vi "get FPGA CD resources.vi"(8 "error in (no error)":errorcluster, 9 "get unmapped?":bool, 10 "get mapped?":bool, 11 "Item Ref in":T2 format="%.0x") -> (0 "error out":errorcluster, 3 "FPGA CD resources":T1[](array[typedef]) {"FPGA CD Ref" format="%.0x"; "reserver" format="%.0x"})   [LabVIEW 2016, in "FPGA Resource Manager System Defintion.lvlib"]
uses:
  FPGA Resource Manager System Defintion.lvlib
  <vilib>/NI Veristand/Custom Device API/Custom Device Item Ref.ctl
  resource info.ctl
  FPGA-Addon/Source/Shared/FG Action.ctl
  global constants.vi
  <vilib>/NI Veristand/Custom Device API/NI VeriStand - Get Item Property.vi
  <vilib>/NI Veristand/Custom Device API/Get Item Property (Variant).vi
  <vilib>/NI Veristand/Custom Device API/NI VeriStand - Set Item Property.vi
  <vilib>/NI Veristand/Custom Device API/Set Item Property (Variant).vi
  <vilib>/NI Veristand/Custom Device API/Custom Device API.lvlib
  FPGA Resource Manager Shared.lvlib
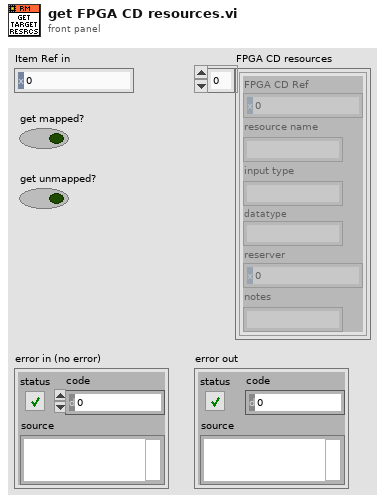
[diagram p1: front panel]
types:
  T1 = typedef "FPGA Resource Manager System Defintion.lvlib/resource info.ctl" = cluster{"FPGA CD Ref":T2, "resource name":string, "input type":string, "datatype":string, "reserver":T2, "notes":string}
  T2 = typedef "Custom Device API.lvlib/Custom Device Item Ref.ctl" = u64
  T3 = typedef "FPGA Resource Manager Shared.lvlib/FG Action.ctl" = enum8{"GET", "SET"}
  T4 = typedef "Custom Device API.lvlib/Custom Device Item Info.ctl" = cluster{"Name":string, "Is Channel":bool, "GUID":string, "Is Waveform":bool}
  T5 = typedef "FPGA Addon Shared.lvlib/Register Information.ctl" = cluster{"Name":string, "Data Type":T6, "Default Value":variant}
  T6 = typedef "FPGA Addon Shared.lvlib/Data Type.ctl" = enum8{"<Null>", "I8", "I16", "I32", "I64", "U8", "U16", "U32", "U64", "SGL", "Boolean", "Analog PWM In Settings", "Analog PWM In", "Digital PWM In Settings", "Digital PWM In", "Digital PWM Out", "Sine Out", "FXP+/-24.5", "FXP+/-16.5", "FXP+/-32.8", "FXP+/-64.32", "FXP+/-16.7", "FXP+/-20.5"}
  T7 = typedef "Fifo_DMA_Config.ctl" = cluster{"Name":string, "Depth":u32, "Write? (Deprecated:Use Implementation)":bool, "Physical Channel":u32, "Base Address":u32, "Data Width":u32, "Data Type":T8, "FXP Properties":variant, "Write Window Address":u32, "Implementation":T9, "Control Set":u32}
  T8 = typedef "niFpgaDataTypeControl.ctl" = enum32{"Boolean", "I8", "I16", "I32", "I64", "U8", "U16", "U32", "U64", "FXP", "CustomControl", "SGL"}
  T9 = typedef "niFpgaDmaChannelImplementation.ctl" = enum16{"niFpgaTargetToHost", "niFpgaHostToTarget", "niFpgaPeerToPeerWriter", "niFpgaPeerToPeerReader", "niCoreTargetToHost", "niCoreHostToTarget"}
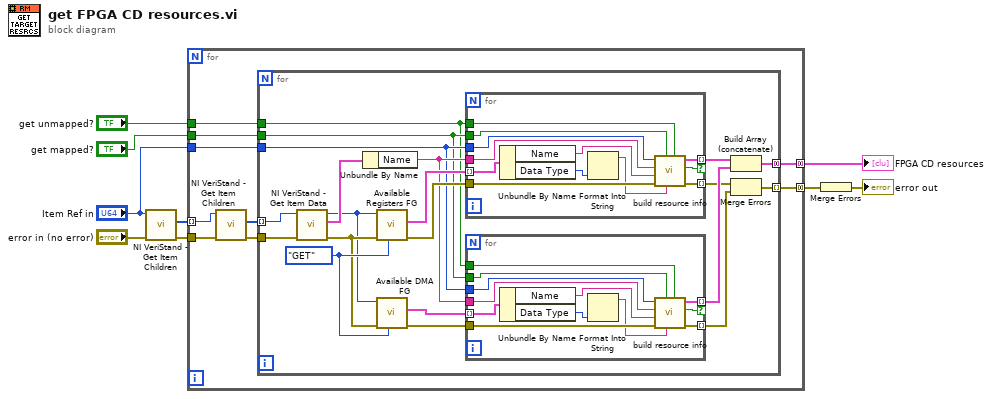
[diagram p0: block diagram]
diagram:
  n1 = call <vilib>:"NI VeriStand - Get Item Children.vi"("error in (no error)"="error in (no error)", "Item Ref in"="Item Ref in") -> ("error out"=w5:errorcluster, "Child Refs"=w6:T2[])  [unwired: 6 in, 2 out]
  n2 = for {
    tunnel: w5 -> [w17]
    tunnel: w6 -> [w15] mode=indexing
    tunnel: "Item Ref in" -> [w14]
    tunnel: [w13] -> w7 mode=concatenating
    tunnel: [w12] -> w2 mode=concatenating
    tunnel: "get mapped?" -> [w11]
    tunnel: "get unmapped?" -> [w10]
    n3 = call <vilib>:"NI VeriStand - Get Item Children.vi"("error in (no error)"=w17, "Item Ref in"=w15) -> ("error out"=w16:errorcluster, "Child Refs"=w18:T2[])  [unwired: 6 in, 2 out]
    n4 = for {
      tunnel: w16 -> [w29]
      tunnel: w18 -> [w32] mode=indexing
      tunnel: w14 -> [w23]
      tunnel: [w36] -> w13 mode=indexing
      tunnel: [w34] -> w12 mode=concatenating
      tunnel: w11 -> [w22]
      tunnel: w10 -> [w21]
      w33 = FG_Action."GET" ("Action")
      n5 = call <vilib>:"NI VeriStand - Get Item Data.vi"("error in (no error)"=w29, "Item Ref in"=w32) -> ("error out"=w28:errorcluster, "Item Info"=w31:T4, "Item Ref out"=w27:T2)  [unwired: 6 in, 1 out]
      n6 = Unbundle By Name(w31) -> ("Name"=w24:string)
      n7 = call "Available Registers FG.vi"("Action"=w33, "error in (no error)"=w28, "Item Ref"=w27) -> ("error out"=w25:errorcluster, "Available Registers"=w26:T5[])  [unwired: 6 in, 1 out]
      n8 = call "Available DMA FG.vi"("Action"=w33, "error in (no error)"=w28, "Item Ref"=w27) -> ("error out"=w30:errorcluster, "Available DMA"=w38:T7[])  [unwired: 6 in, 1 out]
      n9 = for {
        tunnel: w26 -> [w50] mode=indexing
        tunnel: w25 -> [w48]
        tunnel: [w47] -> w19 mode=indexing
        tunnel: [w42] -> w20 mode=indexing if=w49
        tunnel: w22 -> [w46]
        tunnel: w21 -> [w45]
        tunnel: w23 -> [w41]
        tunnel: w24 -> [w40]
        n10 = Unbundle By Name(w50) -> ("Name"=w44:string, "Data Type"=w43:T6)
        n11 = Format Into String(w43) -> (resulting string=w39:string)  [unwired: 3 in, 1 out]
        n12 = call "build resource info.vi"("get unmapped?"=w45, "datatype"=w39, "get mapped?"=w46, "error in (no error)"=w48, "name in bitfile"=w44, "input type"=w40, "FPGA CD Ref"=w41) -> ("error out"=w47:errorcluster, "include?"=w49:bool, "visualizer entry"=w42:T1)  [unwired: 2 in]
      }
      n13 = for {
        tunnel: w38 -> [w62] mode=indexing
        tunnel: w30 -> [w59]
        tunnel: [w58] -> w37 mode=indexing
        tunnel: [w61] -> w35 mode=indexing if=w60
        tunnel: w22 -> [w57]
        tunnel: w21 -> [w56]
        tunnel: w23 -> [w54]
        tunnel: w24 -> [w53]
        n14 = Unbundle By Name(w62) -> ("Name"=w52:string, "Data Type"=w55:T8)
        n15 = Format Into String(w55) -> (resulting string=w51:string)  [unwired: 3 in, 1 out]
        n16 = call "build resource info.vi"("get unmapped?"=w56, "datatype"=w51, "get mapped?"=w57, "error in (no error)"=w59, "name in bitfile"=w52, "input type"=w53, "FPGA CD Ref"=w54) -> ("error out"=w58:errorcluster, "include?"=w60:bool, "visualizer entry"=w61:T1)  [unwired: 2 in]
      }
      n17 = Build Array (concatenate)(w20, w35) -> (w34:T1[])
      n18 = Merge Errors(w19, w37) -> (w36:errorcluster)
    }
  }
  "FPGA CD resources" <- w2
  n19 = Merge Errors(w7) -> (→"error out":errorcluster)
